vi "CODMn启动参数对话框.vi"() -> (1 "标样浓度输出":dbl, 2 "确认":bool, 3 "元素":cluster{"命令":string, "data":variant})   [LabVIEW 2016, in "斯坦道CODMn新电路板.lvlib"]
panel:
  in  "维护模式":bool
  in  "标样浓度":dbl
  in  "取消":bool
  in  "确定":bool
  in  "测量间隔":u16
  in  "模式设置":T1(ring)
  in  "量程切换":enum32{"H", "L", "AUTO"}(radio)=enum."AUTO"
  in  "站号":u16(ring)=21 items=["CODMn"=21]
  in  "控制命令":u16(ring)=1 items=["启动测量"=1, "标样核查"=2, "零点核查"=3, "跨度核查"=4, "空白测试"=5, "平行样测试"=6, "加标回收"=7, "空白校准"=8, "标样校准"=9, "初始化（清洗）"=10, "停止测试"=11, "仪器重启"=12, "校时"=13, "模式设置"=14, "测量间隔设置"=15, "调试"=22, "填充管路"=30, "清洗管路"=31, "清洗反应杯"=32]
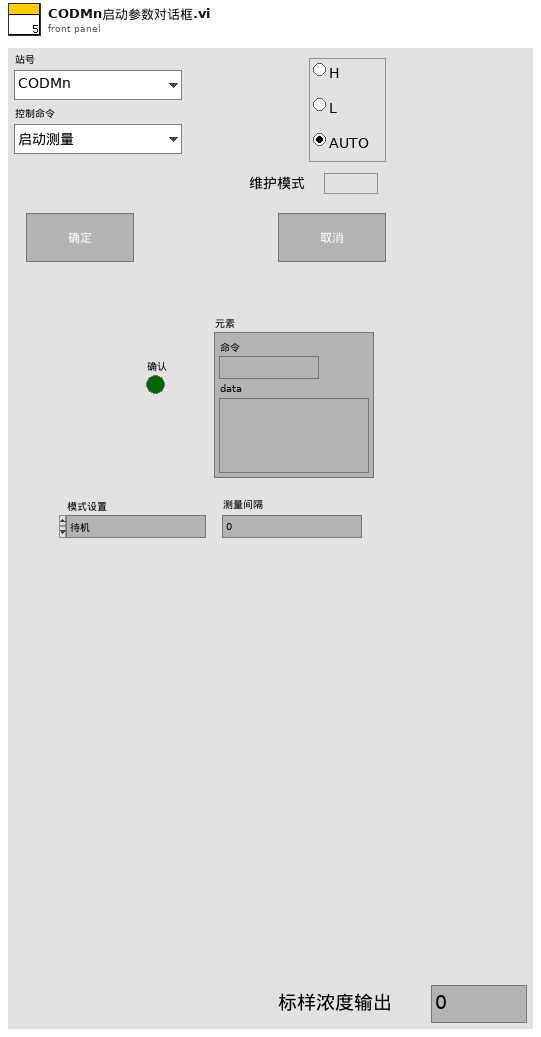
[diagram p1: front panel]
types:
  T1 = enum16{"待机", "连续模式", "周期模式", "定点模式", "受控模式", "手动模式"}
  T2 = cluster{"站号":u16, "量程切换":enum32{"H", "L", "AUTO"}, "控制命令":u16, "模式设置":enum16{"待机", "连续模式", "周期模式", "定点模式", "受控模式", "手动模式"}, "测量间隔":u16}
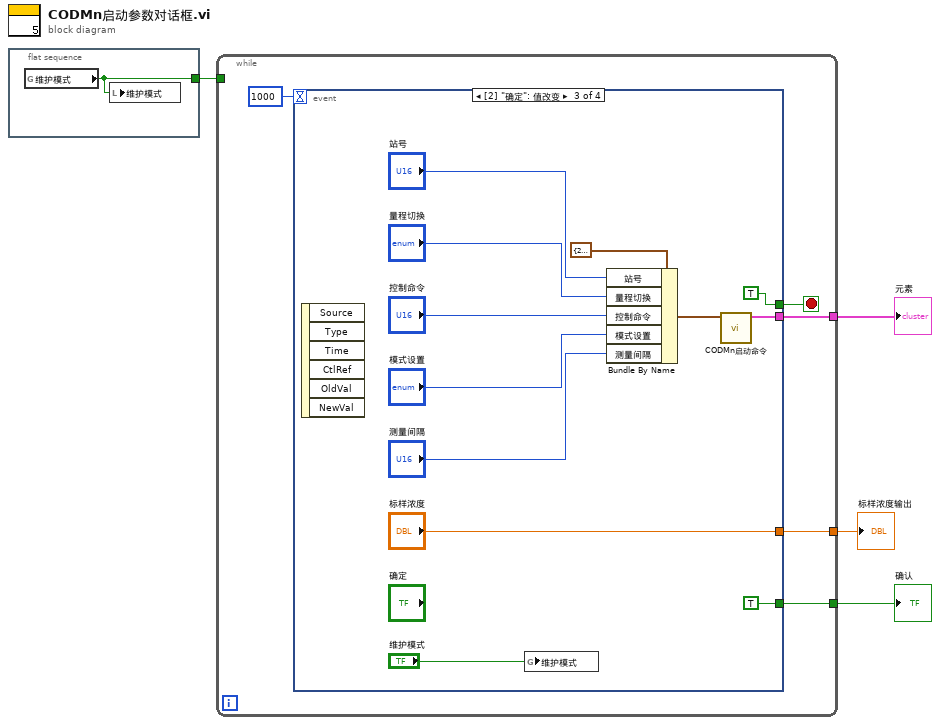
[diagram p0: block diagram]
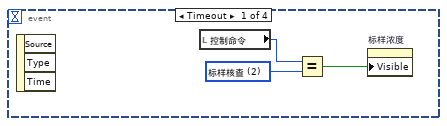
[diagram p2: hidden frame]
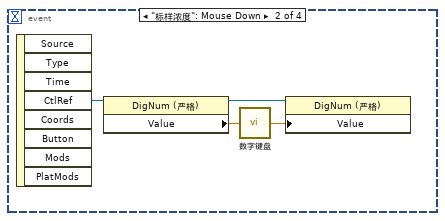
[diagram p3: hidden frame]
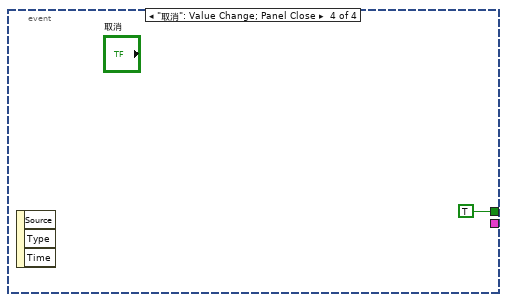
[diagram p4: hidden frame]
diagram:
  n1 = flat-sequence {
    tunnel: [w5] -> w1
    frame #0 {
      n2 = global read "VARCODMn全局变量.vi" "维护模式"() -> (w5:bool)
      n3 = local write "维护模式"(w5) -> ()
    }
  }
  n4 = while {
    tunnel: [w8] -> w4
    tunnel: [w7] -> w3
    tunnel: [w6] -> w2
    tunnel: w1 -> [_]
    stop <- w10 stop-if-true
    n5 = event shown="[2] \"确定\": 值改变" {
      selector: _ -> [_ _ _ _]
      dyn-events: _ -> [_ _ _ _]
      timeout: 1000 -> [_ _ _ _]
      tunnel: [_ _ TRUE TRUE] -> w10
      tunnel: [_ _ TRUE _] -> w8
      tunnel: [_ _ w27 _] -> w7
      tunnel: [_ _ "标样浓度" _] -> w6
      event Timeout {
        w12 = u16 2 items=["启动测量"=1, "标样核查"=2, "零点核查"=3, "跨度核查"=4, "空白测试"=5, "平行样测试"=6, "加标回收"=7, "空白校准"=8, "标样校准"=9, "初始化（清洗）"=10, "停止测试"=11, "仪器重启"=12, "校时"=13, "模式设置"=14, "测量间隔设置"=15, "调试"=22, "填充管路"=30, "清洗管路"=31, "清洗反应杯"=32] ("控制命令")
        n6 = event-data() -> ()  [unwired: 1 in, 3 out]
        n7 = local read "控制命令"() -> (w13:u16)
        n8 = Equal?(x=w13, y=w12) -> (x = y?=w11:bool)
        n9 = property on="标样浓度" class="DigNum (严格)"("Visible"=w11) -> ()  [unwired: 2 in, 2 out]
      }
      event "标样浓度": Mouse Down {
        n10 = event-data() -> ("CtlRef"=w17:refnum<vi>)  [unwired: 1 in, 7 out]
        n11 = property class="DigNum (严格)"(reference=w17) -> (reference out=w16:refnum<vi>, "Value"=w15:dbl)  [unwired: 1 in, 1 out]
        n12 = call "数字键盘.vi"("OldNumber"=w15) -> ("NewNumber"=w14:dbl)
        n13 = property class="DigNum (严格)"(reference=w16, "Value"=w14) -> ()  [unwired: 1 in, 2 out]
      }
      event "确定": Value Change {
        n14 = event-data() -> ()  [unwired: 1 in, 6 out]
        n15 = global write "VARCODMn全局变量.vi" "维护模式"("维护模式") -> ()
        n16 = Bundle By Name(cluster=T2 {"站号"=21, "量程切换"=enum."AUTO", "控制命令"=1, "模式设置"=enum."待机", "测量间隔"=0} ("参数"), "站号"="站号", "量程切换"="量程切换", "控制命令"="控制命令", "模式设置"="模式设置", "测量间隔"="测量间隔") -> (w25:T2)
        n17 = call "CODMn启动命令.vi"("参数"=w25) -> ("启动命令"=w27:cluster{"命令":string, "data":variant})  [unwired: 10 in]
      }
      event "取消": Value Change; Panel Close {
        n18 = event-data() -> ()  [unwired: 1 in, 3 out]
      }
    }
  }
  "元素" <- w3
  "确认" <- w4
  "标样浓度输出" <- w2
